vi "CAT071_main.vi"() -> ()   [LabVIEW 2015]
uses:
  class.dbc/controls/dbc-signal.ctl
  class.dbc/controls/dbc-frame.ctl
  class.dbc/controls/dbc-cluster.ctl
  class.can.table/CAN_table.ctl
  class.dbc/controls/signals.result.ctl
  class.dbc/controls/signal.result.ctl
  subs/frame.type.ctl
  class.bFrameIO/bFrameIO.lvclass/bFrameIO.ctl
  class.dbc/dbc.lvclass/dbc.ctl
  class.bFrameIO/controls/input-states.ctl
  class.dbc/Read-active-frame-tag.vi
  class.dbc/Read-active-item-symbol.vi
  class.dbc/Read-active-item-tag.vi
  class.bFrameIO/wrt-fi-state.vi
  class.dbc/Write-active-item-tag.vi
  class.dbc/Write-active-item-indent-lvl.vi
  class.dbc/Write-active-item-symbol.vi
  class.bFrameIO/wrt-device.vi
  class.bFrameIO/Read-frameQ.vi
  class.bFrameIO/wrt-baud-rate.vi
  class.dbc/dbc.lvclass
  class.bFrameIO/bFrameIO.lvclass
  LEDarray/LEDarray.lvclass
  class.can.table/bAPPdata.lvclass
panel:
  in  "Interface":refnum<k21>
  in  "dbc.alias":string="CAT071"
  out "Path":path caption="Open .dbc file"
  in  "CAT.071":enum32{"DBC", "table"}(tab)
  in  "attributes":T1(tab)
  out "CAN.table":T2
  out "dbc.cluster":T3={"Name"="", "Baud Rate"=125000, "Application Protocol"=enum."None", "Comment"=""}
  out "signal.results":T4 {"payload" format="%3d"}
  out "dbc.frame":T6={"Comment"="", "Extended Identifier?"=FALSE, "Transmit Time"=0.0, "Timing Type"=1, "Payload Length"=8, "Identifier"=1, "Frame name"="frame1"} {"Timing Type" items=["Cyclic Data", "Event Data", "Cyclic Remote", "Event Remote"]; "Identifier" format="%010x"}
  out "payload":bool[][](array[boolean])
  in  "send.frame":bool
  in  "frame.type":T7
  in  "send.signal":bool
  out "leds":picture
  out "output.signal":T8={"Comment"="", "Byte Order"=0, "Data Type"=1, "Number of Bits"=8, "Start Bit"=0, "Unit"="V", "Default Value"=0.0, "Minimum Value"=0.0, "Maximum Value"=256.0, "Scaling Offset"=0.0, "Scaling Factor"=1.0, "Signal name"="signal1"} {"Byte Order" items=["Little Endian", "Big Endian"]; "Data Type" items=["Signed", "Unsigned", "IEEE Float"]}
  out "signal.payload":u32
  in  "hslide":dbl(slide) min=0.0 max=3.0 scale=0.0..3.0
  out "input.signal":T8={"Comment"="", "Byte Order"=0, "Data Type"=1, "Number of Bits"=8, "Start Bit"=0, "Unit"="V", "Default Value"=0.0, "Minimum Value"=0.0, "Maximum Value"=256.0, "Scaling Offset"=0.0, "Scaling Factor"=1.0, "Signal name"="signal1"} {"Byte Order" items=["Little Endian", "Big Endian"]; "Data Type" items=["Signed", "Unsigned", "IEEE Float"]}
  out "signal.payload 2":u32 caption="signal.payload"
  out "payload 2":bool[][](array[boolean]) caption="payload"
  out "nd.signal":T8={"Comment"="", "Byte Order"=0, "Data Type"=1, "Number of Bits"=8, "Start Bit"=0, "Unit"="V", "Default Value"=0.0, "Minimum Value"=0.0, "Maximum Value"=256.0, "Scaling Offset"=0.0, "Scaling Factor"=1.0, "Signal name"="signal1"} {"Byte Order" items=["Little Endian", "Big Endian"]; "Data Type" items=["Signed", "Unsigned", "IEEE Float"]}
  in  "database":string(tree)
  # "CAT 071 \nMarquardt Inc @2017\nK.R. Bergerstock"
  # "CLUSTER"
  # "FRAME"
  # "SIGNAL"
  # "SIGNAL"
  # "SIGNAL"
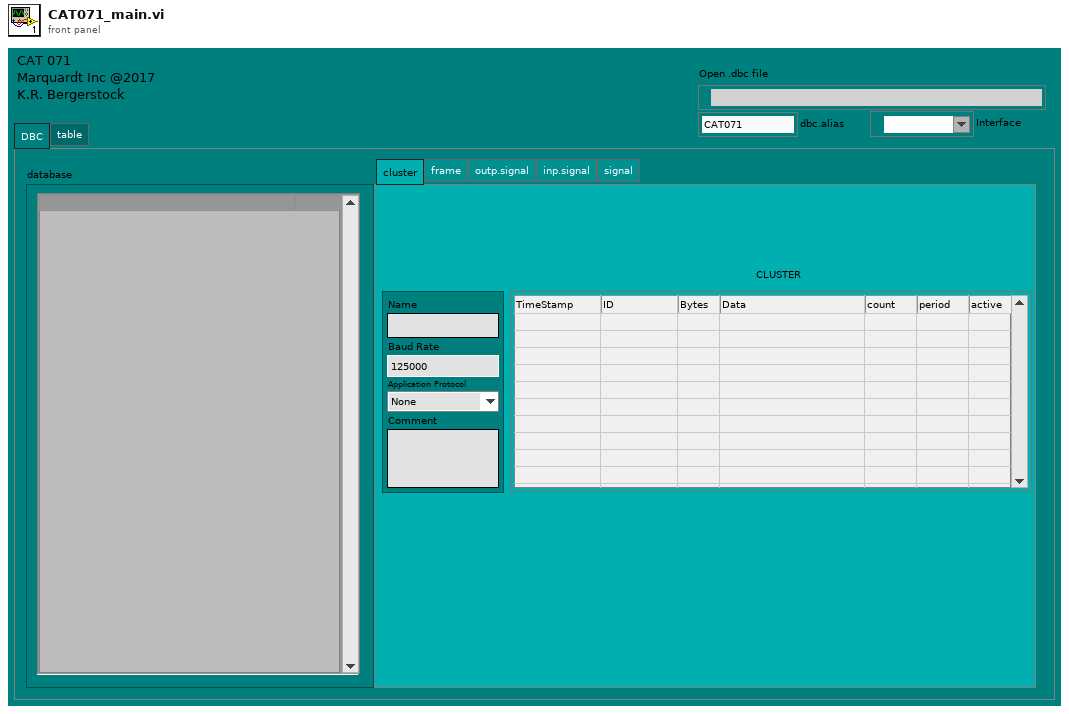
[diagram p1: front panel]
types:
  T1 = enum32{"cluster", "frame", "outp.signal", "inp.signal", "signal"}
  T2 = typedef "CAN_table.ctl" = string[][]
  T3 = typedef "dbc-cluster.ctl" = cluster{"Name":string, "Baud Rate":u32, "Application Protocol":enum16{"None", "J1939"}, "Comment":string}
  T4 = typedef "signals.result.ctl" = T5[]
  T5 = typedef "signal.result.ctl" = cluster{"Signal name":string, "payload":u8}
  T6 = typedef "dbc-frame.ctl" = cluster{"Comment":string, "Extended Identifier?":bool, "Transmit Time":dbl, "Timing Type":u32, "Payload Length":u32, "Identifier":u32, "Frame name":string}
  T7 = typedef "frame.type.ctl" = enum16{"FRAME NOT DEFINED", "DUT OUTPUT FRAME", "DUT INPUT FRAME"}
  T8 = typedef "dbc-signal.ctl" = cluster{"Comment":string, "Byte Order":u32, "Data Type":u32, "Number of Bits":u32, "Start Bit":u32, "Unit":string, "Default Value":dbl, "Minimum Value":dbl, "Maximum Value":dbl, "Scaling Offset":dbl, "Scaling Factor":dbl, "Signal name":string}
  T9 = typedef "bFrameIO.lvclass/input-states.ctl" = enum16{"idle", "start", "run", "stop", "exit"}
  T10 = enum32{"cluster", "frame", "outp.signal", "inp.signal"}
  T11 = typedef "frame-defination.ctl" = cluster{"CAN.frame":T6, "frame.type":T7}
  T12 = typedef "LVPoint32TypeDef.ctl" = cluster{"Horizontal":i32, "Vertical":i32}
  T13 = typedef "LVRectTypeDef.ctl" = cluster{"Left":i16, "Top":i16, "Right":i16, "Bottom":i16}
  T14 = typedef "XNET Frame CAN.ctl" = cluster{"timestamp":timestamp, "payload":u8[], "identifier":u32, "type":T15, "extended?":bool, "echo?":bool}
  T15 = typedef "XNET Frame Type CAN.ctl" = u8
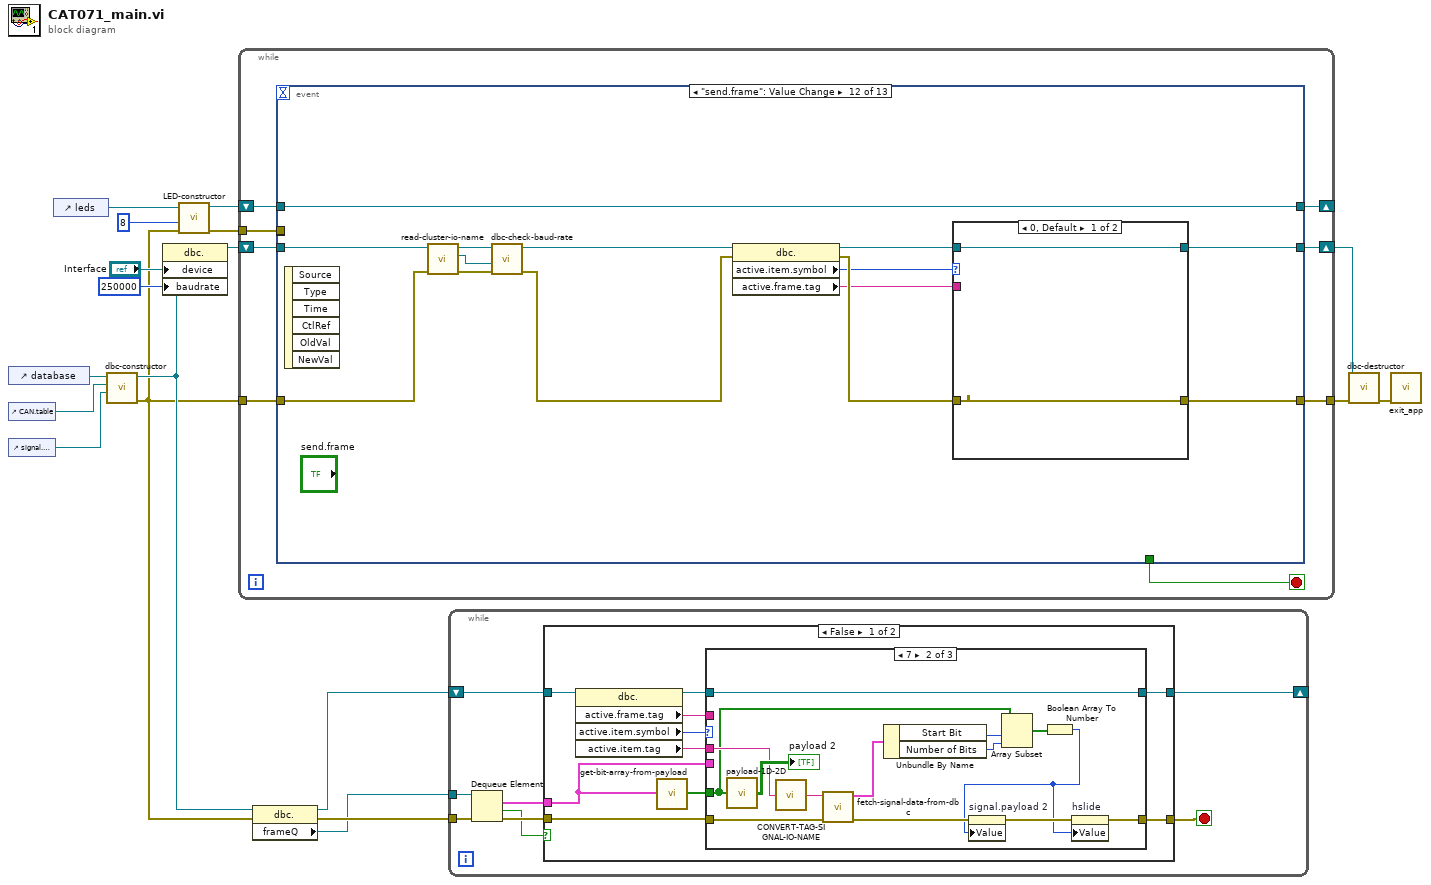
[diagram p0: block diagram]
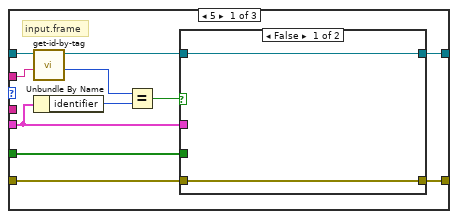
[diagram p2: hidden frame]
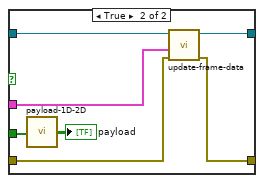
[diagram p3: hidden frame]
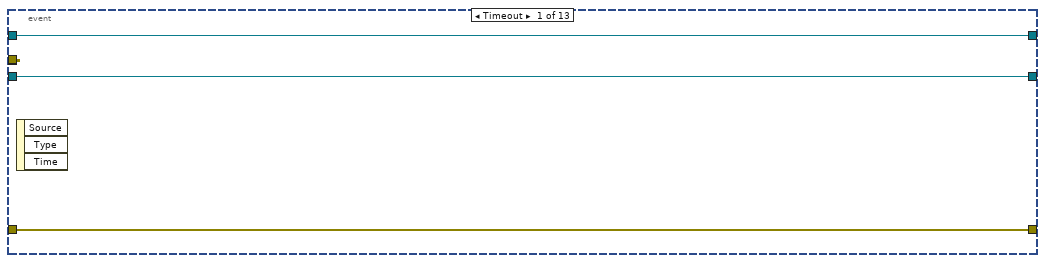
[diagram p6: hidden frame]
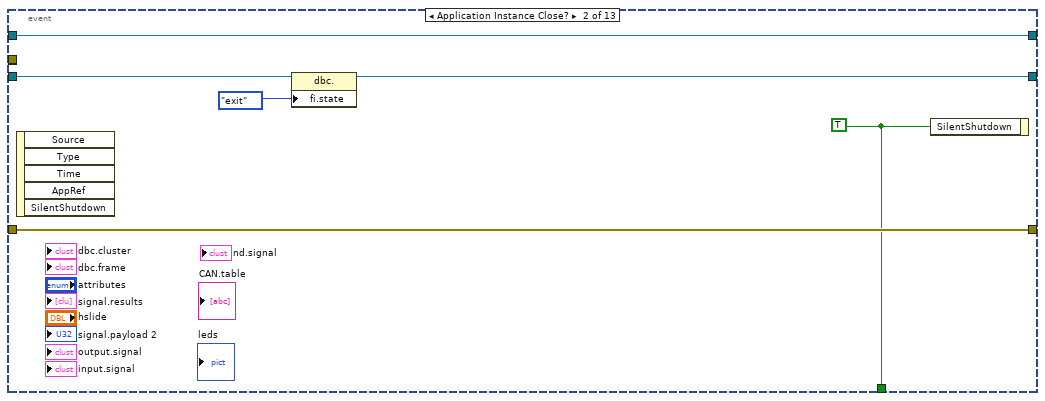
[diagram p7: hidden frame]
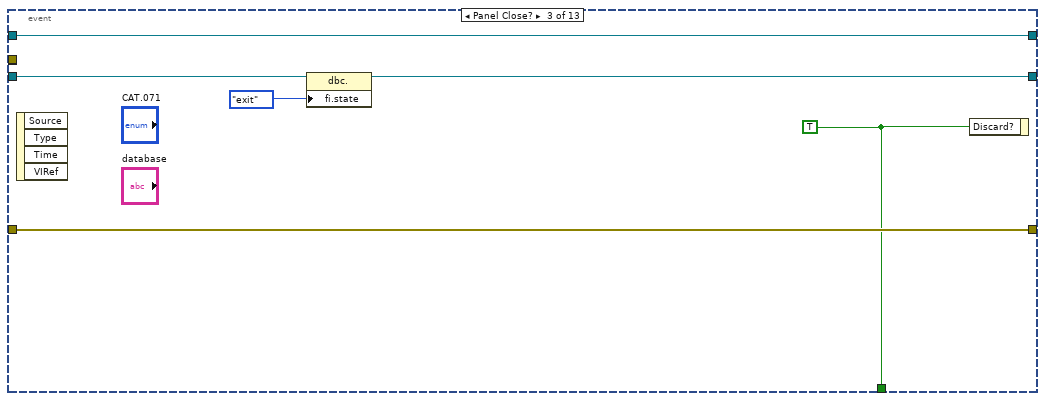
[diagram p8: hidden frame]
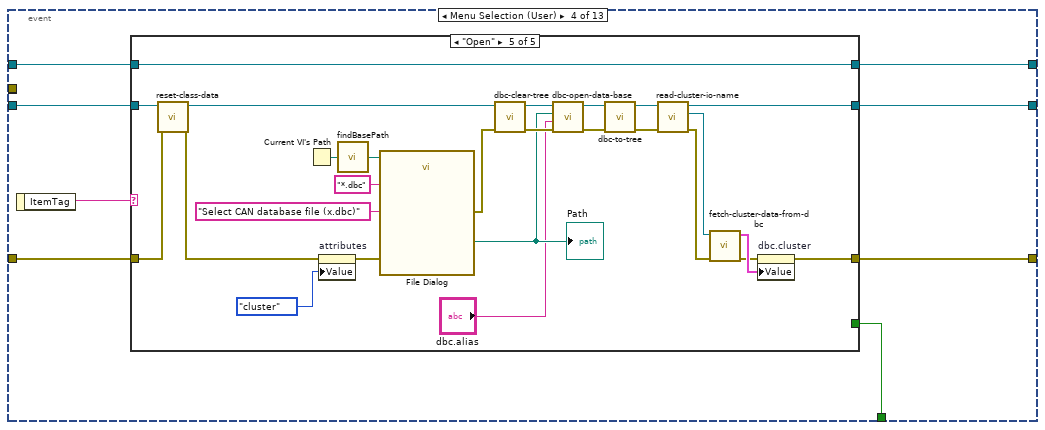
[diagram p9: hidden frame]
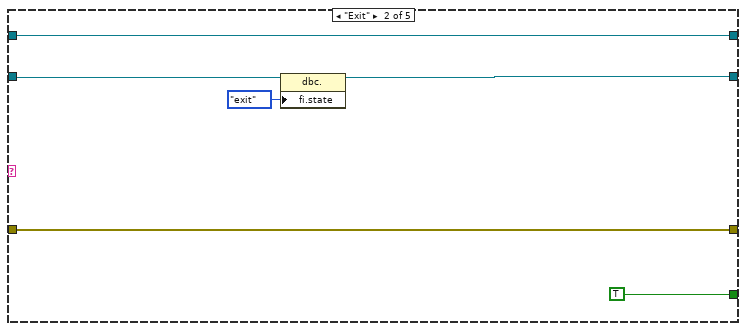
[diagram p11: hidden frame]
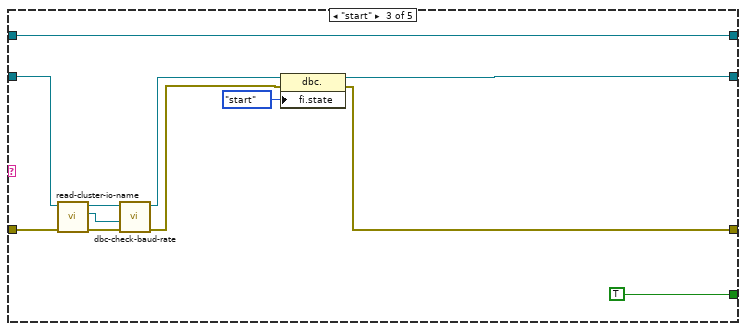
[diagram p12: hidden frame]
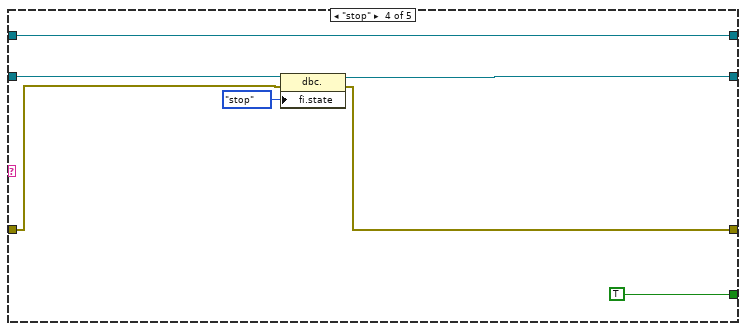
[diagram p13: hidden frame]
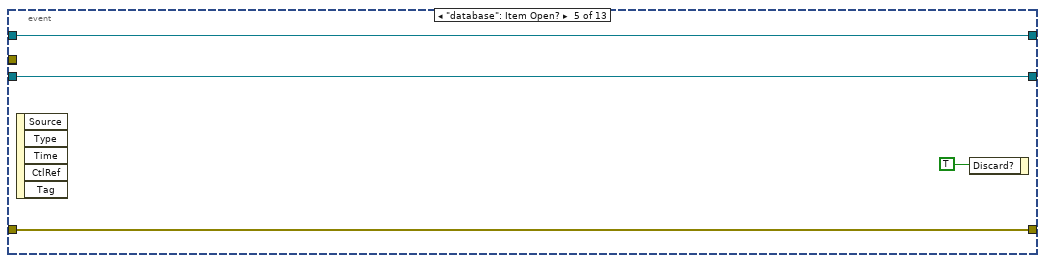
[diagram p14: hidden frame]
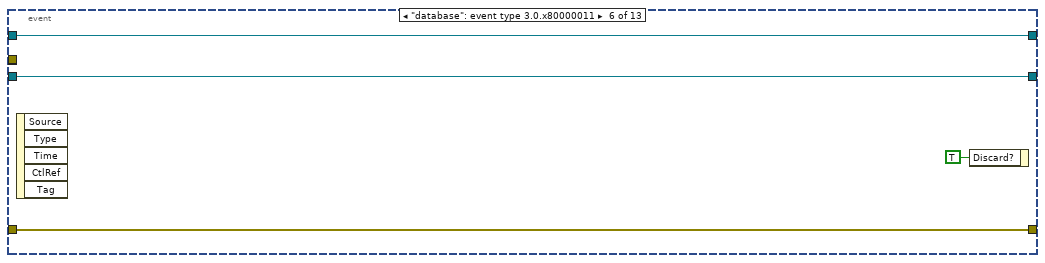
[diagram p15: hidden frame]
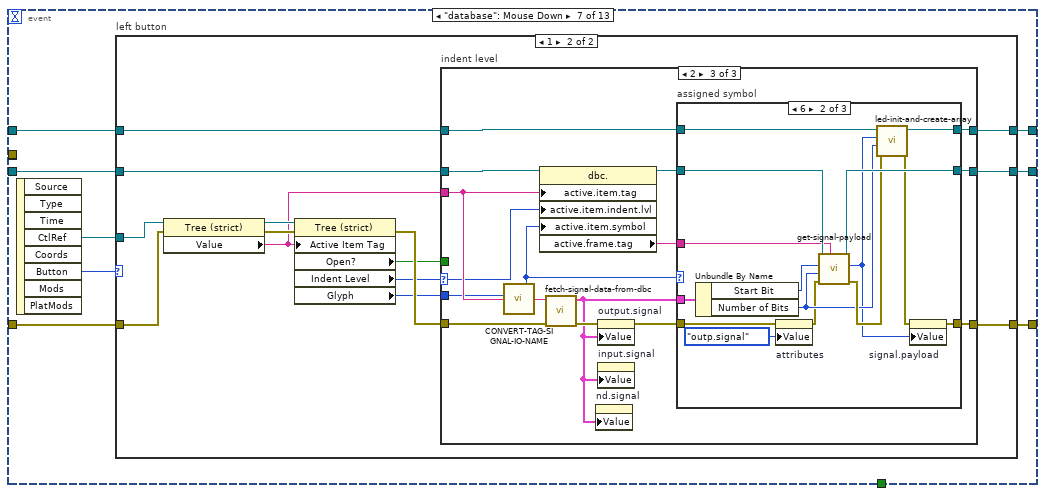
[diagram p16: hidden frame]
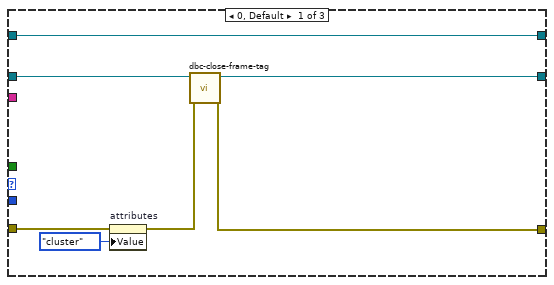
[diagram p18: hidden frame]
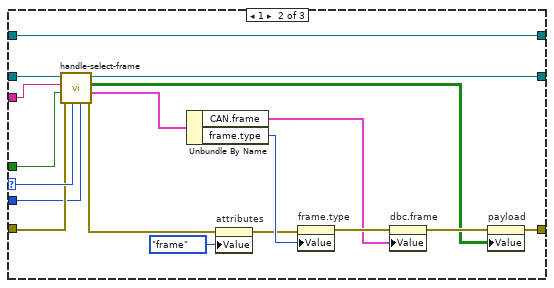
[diagram p19: hidden frame]
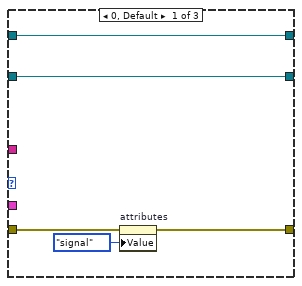
[diagram p20: hidden frame]
diagram:
  n1 = control-ref of="database"() -> (w17:refnum<vi>)
  n2 = control-ref of="CAN.table"() -> (w8:refnum<vi>)
  n3 = control-ref of="signal.results"() -> (w1:refnum<vi>)
  n4 = control-ref of="leds"() -> (w14:refnum<vi>)
  n5 = call "dbc-constructor.vi"("signal.results"=w1, "table.ref in"=w8, "tree.ref.in"=w17) -> ("error out"=w2:errorcluster, "dbc out"=w5:refnum<class "dbc.lvclass">)  [unwired: 7 in]
  n6 = property class="dbc."(reference=w5, "device"="Interface", "baudrate"=u32 250000) -> (reference out=w10:refnum<class "dbc.lvclass">)  [unwired: 1 in, 1 out]
  n7 = call "LED-constructor.vi"("error in (no error)"=w2, "radius"=8, "picture.ref"=w14) -> ("error out"=w11:errorcluster, "LEDarray out"=w12:refnum<class "LEDarray.lvclass">)  [unwired: 7 in]
  n8 = while {
    shift-right: [w19] -> w16
    shift-left: w10 -> [w26]
    tunnel: w2 -> [w25]
    tunnel: [w24] -> w9
    shift-right: [w21] -> _
    shift-left: w12 -> [w22]
    tunnel: w11 -> [w20]
    stop <- w23 stop-if-true
    n9 = event shown="[11] \"send.frame\": Value Change" {
      selector: _ -> [_ _ _ _ _ _ _ _ _ _ _ _ _]
      dyn-events: _ -> [_ _ _ _ _ _ _ _ _ _ _ _ _]
      timeout: _ -> [_ _ _ _ _ _ _ _ _ _ _ _ _]
      tunnel: [w28 w33 w39 w46 w107 w111 w116 w213 w240 w272 w290 w311 w324] -> w19
      tunnel: w26 -> [w28 w36 w42 w47 w107 w111 w115 w214 w241 w272 w282 w305 w327]
      tunnel: w25 -> [w27 w35 w41 w48 w106 w110 w113 w216 w243 w257 w297 w303 w326]
      tunnel: [w27 w35 w41 w49 w106 w110 w114 w215 w242 w259 w287 w310 w326] -> w24
      tunnel: [_ w34 w40 w45 _ _ _ _ _ _ _ _ _] -> w23
      tunnel: w22 -> [w30 w31 w37 w44 w105 w109 w117 w210 w244 w271 w296 w312 w325]
      tunnel: [w30 w31 w37 w43 w105 w109 w118 w211 w244 w261 w296 w312 w325] -> w21
      tunnel: [w29 _ _ _ _ _ _ _ _ _ _ _ _] -> _
      tunnel: w20 -> [w29 _ _ _ _ _ _ _ _ _ _ _ _]
      event Timeout {
        n10 = event-data() -> ()  [unwired: 1 in, 3 out]
      }
      event Application Instance Close? {
        w34 = TRUE
        n11 = event-data() -> ()  [unwired: 1 in, 5 out]
        n12 = property class="dbc."(reference=w36, "fi.state"=input-states."exit") -> (reference out=w33:refnum<class "dbc.lvclass">)  [unwired: 1 in, 1 out]
        n13 = event-data("SilentShutdown"=w34) -> ()  [unwired: 1 in, 1 out]
      }
      event Panel Close? {
        w40 = TRUE
        n14 = event-data() -> ()  [unwired: 1 in, 4 out]
        n15 = property class="dbc."(reference=w42, "fi.state"=input-states."exit") -> (reference out=w39:refnum<class "dbc.lvclass">)  [unwired: 1 in, 1 out]
        n16 = event-data("Discard?"=w40) -> ()  [unwired: 1 in, 1 out]
      }
      event Menu Selection (User) {
        n17 = event-data() -> ("ItemTag"=w50:string)  [unwired: 1 in]
        n18 = case shown="\"Open\"" w50 {
          tunnel: [w53 w59 w60 w72 w93] -> w49
          tunnel: w48 -> [w53 w59 w64 w74 w81]
          tunnel: w47 -> [w52 w58 w63 w73 w82]
          tunnel: [w52 w56 w70 w77 w90] -> w46
          tunnel: [_ TRUE TRUE TRUE _] -> w45
          tunnel: w44 -> [w51 w54 w68 w75 w85]
          tunnel: [w51 w54 w68 w75 w85] -> w43
          frame Default {
          }
          frame "Exit" {
            n19 = property class="dbc."(reference=w58, "fi.state"=input-states."exit") -> (reference out=w56:refnum<class "dbc.lvclass">)  [unwired: 1 in, 1 out]
          }
          frame "start" {
            n20 = call "read-cluster-io-name.vi"("error in (no error)"=w64, "dbc in"=w63) -> ("error out"=w66:errorcluster, "XNET Cluster"=w65:refnum<k21>, "dbc out"=w67:refnum<class "dbc.lvclass">)  [unwired: 7 in]
            n21 = call "dbc-check-baud-rate.vi"("error in (no error)"=w66, "XNET Cluster 2"=w65, "dbc in"=w67) -> ("error out"=w61:errorcluster, "dbc out"=w62:refnum<class "dbc.lvclass">)  [unwired: 7 in]
            n22 = property class="dbc."(reference=w62, error in=w61, "fi.state"=input-states."start") -> (reference out=w70:refnum<class "dbc.lvclass">, error out=w60:errorcluster)
          }
          frame "stop" {
            n23 = property class="dbc."(reference=w73, error in=w74, "fi.state"=input-states."stop") -> (reference out=w77:refnum<class "dbc.lvclass">, error out=w72:errorcluster)
          }
          frame "Open" {
            n24 = call-dynamic "reset-class-data.vi"("error in (no error)"=w81, "CANtable in"=w82) -> ("error out"=w80:errorcluster, "CANtable out"=w84:refnum<class "dbc.lvclass">)  [unwired: 8 in]
            n25 = Current VI's Path() -> (path=w101:path)
            n26 = property on="attributes" class="TabCtl (strict)"(error in=w80, "Value"=T10."cluster" ("attributes")) -> (error out=w86:errorcluster)  [unwired: 1 in, 1 out]
            n27 = call "findBasePath.vi"("path.in"=w101) -> ("path.out"=w100:path)  [unwired: 4 in]
            n28 = call "File Dialog"("start path"=w100, "prompt"="Select CAN database file (x.dbc)", "error in"=w86, "pattern (all files)"="*.dbc") -> ("selected path"=w98:path, "error out"=w103:errorcluster)  [unwired: 8 in, 2 out]
            "Path" <- w98
            n29 = call "dbc-clear-tree.vi"("dbc in"=w84) -> ("dbc out"=w79:refnum<class "dbc.lvclass">)  [unwired: 9 in, 1 out]
            n30 = call "dbc-open-data-base.vi"("error in (no error)"=w103, "alias"="dbc.alias", "dbc.path"=w98, "dbc in"=w79) -> ("error out"=w94:errorcluster, "dbc out"=w99:refnum<class "dbc.lvclass">)  [unwired: 6 in]
            n31 = call "dbc-to-tree.vi"("error in (no error)"=w94, "dbc in"=w99) -> ("error out"=w88:errorcluster, "dbc out"=w95:refnum<class "dbc.lvclass">)  [unwired: 8 in]
            n32 = call "read-cluster-io-name.vi"("error in (no error)"=w88, "dbc in"=w95) -> ("error out"=w87:errorcluster, "XNET Cluster"=w89:refnum<k21>, "dbc out"=w90:refnum<class "dbc.lvclass">)  [unwired: 7 in]
            n33 = call "fetch-cluster-data-from-dbc.vi"("error in (no error)"=w87, "CLUSTER.TAG"=w89) -> ("error out"=w91:errorcluster, "CAN Cluster"=w92:T3)  [unwired: 8 in]
            n34 = property on="dbc.cluster" class="Clust (strict)"(error in=w91, "Value"=w92) -> (error out=w93:errorcluster)  [unwired: 1 in, 1 out]
          }
        }
      }
      event "database": Item Open? {
        n35 = event-data() -> ()  [unwired: 1 in, 5 out]
        n36 = event-data("Discard?"=TRUE) -> ()  [unwired: 1 in, 1 out]
      }
      event "database": event type 3.0.x80000011 {
        n37 = event-data() -> ()  [unwired: 1 in, 5 out]
        n38 = event-data("Discard?"=TRUE) -> ()  [unwired: 1 in, 1 out]
      }
      event "database": Mouse Down {
        n39 = event-data() -> ("CtlRef"=w119:refnum<vi>, "Button"=w112:u16)  [unwired: 1 in, 6 out]
        n40 = case "left button" shown="1" w112 {
          tunnel: w119 -> [_ w136]
          tunnel: [w122 w134] -> w118
          tunnel: w117 -> [w122 w133]
          tunnel: [w121 w132] -> w116
          tunnel: w115 -> [w121 w131]
          tunnel: [w120 w130] -> w114
          tunnel: w113 -> [w120 w128]
          frame 0, Default {
          }
          frame 1 {
            n41 = property class="Tree (strict)"(reference=w136, error in=w128) -> (reference out=w135:refnum<vi>, error out=w129:errorcluster, "Value"=w126:string)
            n42 = property class="Tree (strict)"(reference=w135, error in=w129, "Active Item Tag"=w126) -> (error out=w127:errorcluster, "Open?"=w123:bool, "Indent Level"=w125:i32, "Glyph"=w124:i32)  [unwired: 1 out]
            n43 = case "indent level" shown="2" w125 {
              selector: w125 -> [_ w158 w162]
              tunnel: [w143 w161 w170] -> w134
              tunnel: w133 -> [w143 w161 w171]
              tunnel: [w141 w159 w169] -> w132
              tunnel: w131 -> [w142 w160 w172]
              tunnel: [w139 w156 w168] -> w130
              tunnel: w127 -> [w140 w157 w167]
              tunnel: w126 -> [_ w145 w166]
              tunnel: w124 -> [_ w155 w163]
              tunnel: w123 -> [_ w144 _]
              frame 0, Default {
                n44 = property on="attributes" class="TabCtl (strict)"(error in=w140, "Value"=T1."cluster" ("attributes")) -> (error out=w138:errorcluster)  [unwired: 1 in, 1 out]
                n45 = call "dbc-close-frame-tag.vi"("error in (no error)"=w138, "dbc in"=w142) -> ("error out"=w139:errorcluster, "dbc out"=w141:refnum<class "dbc.lvclass">)  [unwired: 8 in]
              }
              frame 1 {
                n46 = call "handle-select-frame.vi"("symbol"=w155, "Indent Level"=w158, "error in (no error)"=w157, "open?"=w144, "Tag"=w145, "dbc in"=w160) -> ("error out"=w148:errorcluster, "frame.def"=w151:T11, "payload"=w153:bool[][], "dbc out"=w159:refnum<class "dbc.lvclass">)  [unwired: 2 in]
                n47 = Unbundle By Name(w151) -> ("CAN.frame"=w150:T6, "frame.type"=w149:T7)
                n48 = property on="attributes" class="TabCtl (strict)"(error in=w148, "Value"=T1."frame" ("attributes")) -> (error out=w147:errorcluster)  [unwired: 1 in, 1 out]
                n49 = property on="frame.type" class="Enum (strict)"(error in=w147, "Value"=w149) -> (error out=w152:errorcluster)  [unwired: 1 in, 1 out]
                n50 = property on="dbc.frame" class="Clust (strict)"(error in=w152, "Value"=w150) -> (error out=w154:errorcluster)  [unwired: 1 in, 1 out]
                n51 = property on="payload" class="Arr (strict)"(error in=w154, "Value"=w153) -> (error out=w156:errorcluster)  [unwired: 1 in, 1 out]
              }
              frame 2 {
                n52 = call "CONVERT-TAG-SIGNAL-IO-NAME.vi"("tag"=w166) -> ("signal"=w173:string)  [unwired: 4 in]
                n53 = property class="dbc."(reference=w172, "active.item.tag"=w166, "active.item.indent.lvl"=w162, "active.item.symbol"=w163) -> (reference out=w175:refnum<class "dbc.lvclass">, "active.frame.tag"=w174:string)  [unwired: 1 in, 1 out]
                n54 = call "fetch-signal-data-from-dbc.vi"("error in (no error)"=w167, "signal.tag"=w173) -> ("error out"=w176:errorcluster, "can.signal"=w164:T8)  [unwired: 8 in]
                n55 = property on="nd.signal" class="Clust (strict)"("Value"=w164) -> ()  [unwired: 2 in, 2 out]
                n56 = property on="output.signal" class="Clust (strict)"(error in=w176, "Value"=w164) -> (error out=w165:errorcluster)  [unwired: 1 in, 1 out]
                n57 = property on="input.signal" class="Clust (strict)"("Value"=w164) -> ()  [unwired: 2 in, 2 out]
                n58 = case "assigned symbol" shown="6" w163 {
                  tunnel: w164 -> [_ w193 w200]
                  tunnel: w165 -> [w181 w191 w204]
                  tunnel: [w178 w185 w202] -> w168
                  tunnel: [w180 w192 w201] -> w169
                  tunnel: w175 -> [w180 w196 w201]
                  tunnel: [w179 w194 w205] -> w170
                  tunnel: w171 -> [w179 w195 w205]
                  tunnel: w174 -> [_ w189 _]
                  frame 0, Default {
                    n59 = property on="attributes" class="TabCtl (strict)"(error in=w181, "Value"=T1."signal" ("attributes")) -> (error out=w178:errorcluster)  [unwired: 1 in, 1 out]
                  }
                  frame 6 {
                    n60 = Unbundle By Name(w193) -> ("Start Bit"=w188:u32, "Number of Bits"=w187:u32)
                    n61 = property on="attributes" class="TabCtl (strict)"(error in=w191, "Value"=T10."outp.signal" ("attributes")) -> (error out=w183:errorcluster)  [unwired: 1 in, 1 out]
                    n62 = call "get-signal-payload.vi"("frame.tag"=w189, "error in (no error)"=w183, "bit.len"=w187, "start.pos"=w188, "CANtable in"=w196) -> ("error out"=w190:errorcluster, "payload"=w184:u32, "CANtable out"=w192:refnum<class "dbc.lvclass">)  [unwired: 4 in]
                    n63 = call "led-init-and-create-array.vi"("error in (no error)"=w190, "len.bits"=w187, "init.value"=w184, "LEDarray"=w195) -> ("error out"=w186:errorcluster, "LEDarray 2"=w194:refnum<class "LEDarray.lvclass">)  [unwired: 6 in]
                    n64 = property on="signal.payload" class="DigNum (strict)"(error in=w186, "Value"=w184) -> (error out=w185:errorcluster)  [unwired: 1 in, 1 out]
                  }
                  frame 7 {
                    n65 = Unbundle By Name(w200) -> ("Maximum Value"=w198:dbl, "Minimum Value"=w197:dbl)
                    n66 = property on="attributes" class="TabCtl (strict)"(error in=w204, "Value"=T10."inp.signal" ("attributes")) -> (error out=w203:errorcluster)  [unwired: 1 in, 1 out]
                    n67 = property on="hslide" class="Slide (strict)"(error in=w203, "Maximum"=w198, "Scale.Maximum"=w198, "Minimum"=w197, "Scale.Minimum"=w197) -> (error out=w202:errorcluster)  [unwired: 1 in, 1 out]
                  }
                }
              }
            }
          }
        }
      }
      event "database": Double Click {
        n68 = event-data() -> ("CtlRef"=w212:refnum<vi>)  [unwired: 1 in, 6 out]
        n69 = property class="Tree (strict)"(reference=w212, error in=w216) -> (reference out=w218:refnum<vi>, error out=w217:errorcluster, "Value"=w209:string)
        n70 = property class="Tree (strict)"(reference=w218, error in=w217, "Active Item Tag"=w209) -> (error out=w207:errorcluster, "Indent Level"=w208:i32, "Open?"=w206:bool)  [unwired: 1 out]
        n71 = case "indent level" shown="Default" w208 {
          tunnel: w207 -> [w221 w227]
          tunnel: [w221 w225] -> w215
          tunnel: w214 -> [w220 w228]
          tunnel: [w220 w226] -> w213
          tunnel: [w219 w224] -> w211
          tunnel: w210 -> [w219 w223]
          tunnel: w206 -> [_ w222]
          frame Default {
          }
          frame 1 {
            n72 = case "open/close state of tag" shown="False" w222 {
              tunnel: w228 -> [w233 w236]
              tunnel: w227 -> [w232 w234]
              tunnel: [w231 w236] -> w226
              tunnel: [w230 w234] -> w225
              tunnel: [w229 w235] -> w224
              tunnel: w223 -> [w229 w235]
              frame False {
                n73 = call "dbc-open-frame-tag.vi"("error in (no error)"=w232, "dbc in"=w233) -> ("error out"=w230:errorcluster, "dbc out"=w231:refnum<class "dbc.lvclass">)  [unwired: 8 in]
              }
              frame True {
              }
            }
          }
        }
      }
      event Value Change {
        n74 = event-data() -> ("OldVal"=w239:T7, "NewVal"=w237:T7)  [unwired: 1 in, 4 out]
        n75 = Not Equal?(x=w239, y=w237) -> (x != y?=w238:bool)
        n76 = case shown="True" w238 {
          tunnel: w243 -> [w245 w254]
          tunnel: [w245 w253] -> w242
          tunnel: w241 -> [w246 w252]
          tunnel: [w246 w251] -> w240
          tunnel: w237 -> [_ w247]
          frame False {
          }
          frame True {
            n77 = property class="dbc."(reference=w252) -> (reference out=w250:refnum<class "dbc.lvclass">, "active.frame.tag"=w249:string)  [unwired: 1 in, 1 out]
            n78 = property on="dbc.frame" class="Clust (strict)"(error in=w254) -> (error out=w255:errorcluster, "Value"=w248:T6)  [unwired: 1 in, 1 out]
            n79 = call "dbc-mark-frame.vi"("CAN.frame"=w248, "tag"=w249, "error in (no error)"=w255, "action"=w247, "dbc in"=w250) -> ("error out"=w253:errorcluster, "dbc out"=w251:refnum<class "dbc.lvclass">)  [unwired: 5 in]
          }
        }
      }
      event "leds": Mouse Down {
        n80 = event-data() -> ("Coords"=w265:T12, "CtlRef"=w263:refnum<vi>)  [unwired: 1 in, 4 out]
        n81 = property class="Pict"(reference=w263, error in=w257) -> (error out=w256:errorcluster, "MasterRect"=w262:T13)  [unwired: 1 out]
        n82 = call "LED-get-location.vi"("error in (no error)"=w256, "MasterRect"=w262, "Coords"=w265, "LEDarray"=w271) -> ("error out"=w266:errorcluster, "y"=w267:i32, "x"=w268:i32, "LEDarray.out"=w270:refnum<class "LEDarray.lvclass">)  [unwired: 4 in]
        n83 = call "led-change-color.vi"("Color Box"=u32 3524608, "error in (no error)"=w266, "y"=w267, "x"=w268, "LEDarray"=w270) -> ("error out"=w260:errorcluster, "LEDarray 2"=w269:refnum<class "LEDarray.lvclass">)  [unwired: 5 in]
        n84 = call "LED-read-U32.vi"("error in (no error)"=w260, "LEDarray in"=w269) -> ("error out"=w259:errorcluster, "Numeric"=→"signal.payload":u32, "LEDarray out"=w261:refnum<class "LEDarray.lvclass">)  [unwired: 6 in, 1 out]
      }
      event "send.signal": Value Change {
        n85 = event-data() -> ()  [unwired: 1 in, 6 out]
        n86 = property on=".signal" class="Clust (strict)"(error in=w297) -> (error out=w275:errorcluster, "Value"=w295:T8)  [unwired: 1 in, 1 out]
        n87 = Unbundle By Name(w295) -> ("Number of Bits"=w279:u32, "Start Bit"=w280:u32)
        n88 = call "read-cluster-io-name.vi"("error in (no error)"=w275, "dbc in"=w282) -> ("error out"=w285:errorcluster, "XNET Cluster"=w284:refnum<k21>, "dbc out"=w286:refnum<class "dbc.lvclass">)  [unwired: 7 in]
        n89 = call "dbc-check-baud-rate.vi"("error in (no error)"=w285, "XNET Cluster 2"=w284, "dbc in"=w286) -> ("error out"=w274:errorcluster, "dbc out"=w283:refnum<class "dbc.lvclass">)  [unwired: 7 in]
        n90 = property on="signal.payload" class="DigNum (strict)"(error in=w274) -> (error out=w277:errorcluster, "Value"=w276:u32)  [unwired: 1 in, 1 out]
        n91 = Number To Boolean Array(number=w276) -> (Boolean array=w294:bool[])
        n92 = Reshape Array(w294, w279) -> (w278:bool[])
        n93 = property class="dbc."(reference=w283, error in=w277) -> (reference out=w281:refnum<class "dbc.lvclass">, error out=w298:errorcluster, "active.frame.tag"=w273:string)
        n94 = call "update-bit-payload-by-tag.vi"("CANtable in"=w281, "frame.tag"=w273, "Array"=w278, "start.pos"=w280, "error in (no error)"=w298) -> ("CANtable out"=w293:refnum<class "dbc.lvclass">, "error out"=w291:errorcluster)  [unwired: 9 in]
        n95 = call "get-new-can-frame-by-tag.vi"("error in (no error)"=w291, "tag"=w273, "CANtable in"=w293) -> ("error out"=w289:errorcluster, "CAN frame"=w288:T14, "CANtable out"=w292:refnum<class "dbc.lvclass">)  [unwired: 5 in, 1 out]
        n96 = call "output-frame.vi"("error in (no error)"=w289, "CAN frame"=w288, "fi in"=w292) -> ("error out"=w287:errorcluster, "fi out"=w290:refnum<class "dbc.lvclass">)  [unwired: 7 in]
      }
      event "send.frame": Value Change {
        n97 = event-data() -> ()  [unwired: 1 in, 6 out]
        n98 = call "read-cluster-io-name.vi"("error in (no error)"=w303, "dbc in"=w305) -> ("error out"=w308:errorcluster, "XNET Cluster"=w307:refnum<k21>, "dbc out"=w309:refnum<class "dbc.lvclass">)  [unwired: 7 in]
        n99 = call "dbc-check-baud-rate.vi"("error in (no error)"=w308, "XNET Cluster 2"=w307, "dbc in"=w309) -> ("error out"=w302:errorcluster, "dbc out"=w306:refnum<class "dbc.lvclass">)  [unwired: 7 in]
        n100 = property class="dbc."(reference=w306, error in=w302) -> (reference out=w304:refnum<class "dbc.lvclass">, error out=w301:errorcluster, "active.item.symbol"=w299:i32, "active.frame.tag"=w300:string)
        n101 = case shown="0, Default" w299 {
          tunnel: [w314 w321] -> w311
          tunnel: [w313 w318] -> w310
          tunnel: w304 -> [w314 w317]
          tunnel: w301 -> [w313 w316]
          tunnel: w300 -> [_ w315]
          frame 0, Default {
          }
          frame 6 {
            n102 = call "get-new-can-frame-by-tag.vi"("error in (no error)"=w316, "tag"=w315, "CANtable in"=w317) -> ("error out"=w320:errorcluster, "CAN frame"=w319:T14, "CANtable out"=w322:refnum<class "dbc.lvclass">)  [unwired: 5 in, 1 out]
            n103 = call "output-frame.vi"("error in (no error)"=w320, "CAN frame"=w319, "fi in"=w322) -> ("error out"=w318:errorcluster, "fi out"=w321:refnum<class "dbc.lvclass">)  [unwired: 7 in]
          }
        }
      }
      event "Interface": Value Change {
        n104 = event-data() -> ("NewVal"=w323:refnum<k21>)  [unwired: 1 in, 5 out]
        n105 = property class="dbc."(reference=w327, "device"=w323) -> (reference out=w324:refnum<class "dbc.lvclass">)  [unwired: 1 in, 1 out]
      }
    }
  }
  n106 = property class="dbc."(reference=w5, error in=w2) -> (reference out=w4:refnum<class "dbc.lvclass">, error out=w18:errorcluster, "frameQ"=w3:refnum<queue>)
  n107 = while {
    tunnel: w3 -> [w334]
    tunnel: w18 -> [w329]
    shift-right: [w328] -> _
    shift-left: w4 -> [w335]
    stop <- w331 stop-if-true
    n108 = Dequeue Element(queue=w334, error in (no error)=w329) -> (element=w333:T14, timed out?=w330:bool, error out=w332:errorcluster)  [unwired: 1 in, 1 out]
    n109 = case shown="False" w330 {
      tunnel: [w345 w383] -> w331
      tunnel: w332 -> [w344 w383]
      tunnel: w333 -> [w338 _]
      tunnel: w335 -> [w343 w382]
      tunnel: [w342 w382] -> w328
      frame False {
        n110 = property class="dbc."(reference=w343) -> (reference out=w341:refnum<class "dbc.lvclass">, "active.frame.tag"=w339:string, "active.item.symbol"=w340:i32, "active.item.tag"=w336:string)  [unwired: 1 in, 1 out]
        n111 = call "get-bit-array-from-payload.vi"("CAN frame"=w338) -> ("Array"=w337:bool[])  [unwired: 4 in]
        n112 = case shown="7" w340 {
          tunnel: [w354 w376 w381] -> w345
          tunnel: w344 -> [w353 w373 w381]
          tunnel: w337 -> [w352 w370 _]
          tunnel: w338 -> [w347 _ _]
          tunnel: w341 -> [w356 w379 w380]
          tunnel: [w355 w379 w380] -> w342
          tunnel: w339 -> [w350 _ _]
          tunnel: w336 -> [_ w375 _]
          frame 5 {
            # "input.frame"
            n113 = call "get-id-by-tag.vi"("tag"=w350, "CANtable in"=w356) -> ("id"=w348:u32, "CANtable out"=w351:refnum<class "dbc.lvclass">)  [unwired: 7 in, 1 out]
            n114 = Unbundle By Name(w347) -> ("identifier"=w346:u32)
            n115 = Equal?(x=w348, y=w346) -> (x = y?=w349:bool)
            n116 = case shown="False" w349 {
              tunnel: [w357 w364] -> w355
              tunnel: [w358 w363] -> w354
              tunnel: w353 -> [w358 w362]
              tunnel: w352 -> [_ w361]
              tunnel: w347 -> [_ w360]
              tunnel: w351 -> [w357 w359]
              frame False {
              }
              frame True {
                n117 = call "payload-1D-2D.vi"("Array"=w361) -> ("Array 2"=→"payload":bool[][])  [unwired: 4 in]
                n118 = call "update-frame-data.vi"("error in (no error)"=w362, "id"=w360, "dbc in"=w359) -> ("error out"=w363:errorcluster, "dbc out"=w364:refnum<class "dbc.lvclass">)  [unwired: 6 in, 1 out]
              }
            }
          }
          frame 7 {
            n119 = call "payload-1D-2D.vi"("Array"=w370) -> ("Array 2"=→"payload 2":bool[][])  [unwired: 4 in]
            n120 = call "CONVERT-TAG-SIGNAL-IO-NAME.vi"("tag"=w375) -> ("signal"=w374:string)  [unwired: 4 in]
            n121 = call "fetch-signal-data-from-dbc.vi"("error in (no error)"=w373, "signal.tag"=w374) -> ("error out"=w372:errorcluster, "can.signal"=w371:T8)  [unwired: 8 in]
            n122 = Unbundle By Name(w371) -> ("Start Bit"=w369:u32, "Number of Bits"=w368:u32)
            n123 = Array Subset(array=w370, index=w369, length=w368) -> (w367:bool[])
            n124 = Boolean Array To Number(Boolean array=w367) -> (number=w366:u32)
            n125 = property on="signal.payload 2" class="DigNum (strict)"(error in=w372, "Value"=w366) -> (error out=w377:errorcluster)  [unwired: 1 in, 1 out]
            n126 = property on="hslide" class="Slide (strict)"(error in=w377, "Value"=w366) -> (error out=w376:errorcluster)  [unwired: 1 in, 1 out]
          }
          frame Default {
          }
        }
      }
      frame True {
      }
    }
  }
  n127 = call "dbc-destructor.vi"("error in (no error)"=w9, "dbc in"=w16) -> ("error out"=w15:errorcluster)  [unwired: 9 in]
  n128 = call "exit_app.vi"("error in (no error)"=w15) -> ()  [unwired: 11 in]
